vi "LM3Sxxxx_QEI_Config.vi"(8 "error in (no error)":errorcluster, 10 "Config Data":string[](array[string]), 11 "Interrupt Name":string) -> (0 "error out":errorcluster, 3 "Interrupt Configuration":string[](array[string]))   [LabVIEW 2011]
panel:
  in  "Phase error interrupt":bool
  in  "Direction change interrupt":bool
  in  "Index pulse interrupt":bool
  in  "Timer expire interrupt":bool
  in  "Period (ms)":u32=10
  in  "Velocity divider":u32(ring) items=["/1"=0, "/2"=64, "/4"=128, "/8"=192, "/16"=256, "/32"=320, "/64"=384, "/128"=448]
  in  "Enable":bool
  in  "Reset on index pulse":bool=TRUE
  in  "Maximum position":u32=1000
  in  "help":bool
  in  "Swap channel inputs":bool
  in  "Signal mode":u32(ring)=1 items=["Quadrature phase"=1, "Clock and direction"=0]
  in  "cancel":bool
  in  "ok":bool
  in  "Quadrature update mode":u32(ring)=1 items=["Capture A and B"=1, "Capture A only"=0]
  # "Input"
  # "Position"
  # "Velocity"
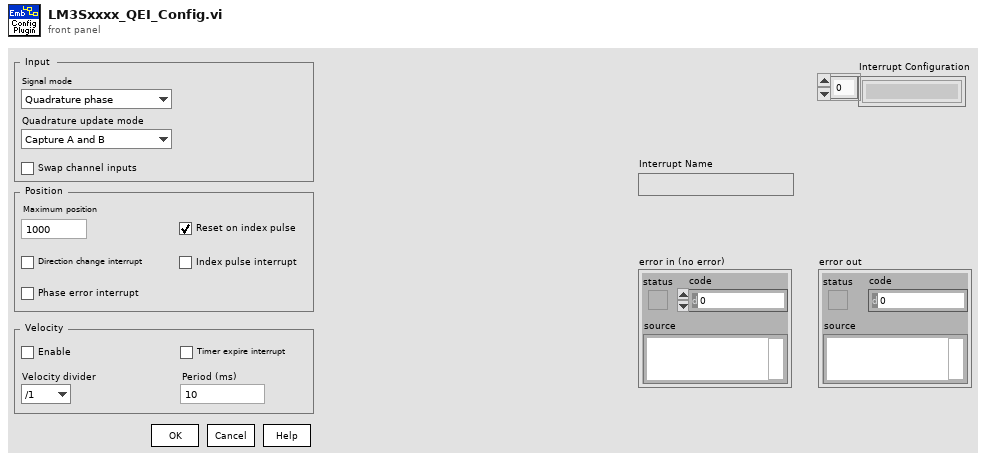
[diagram p1: front panel]
types:
  T1 = enum8{"Enabled", "Disabled", "Disabled and Grayed Out"}
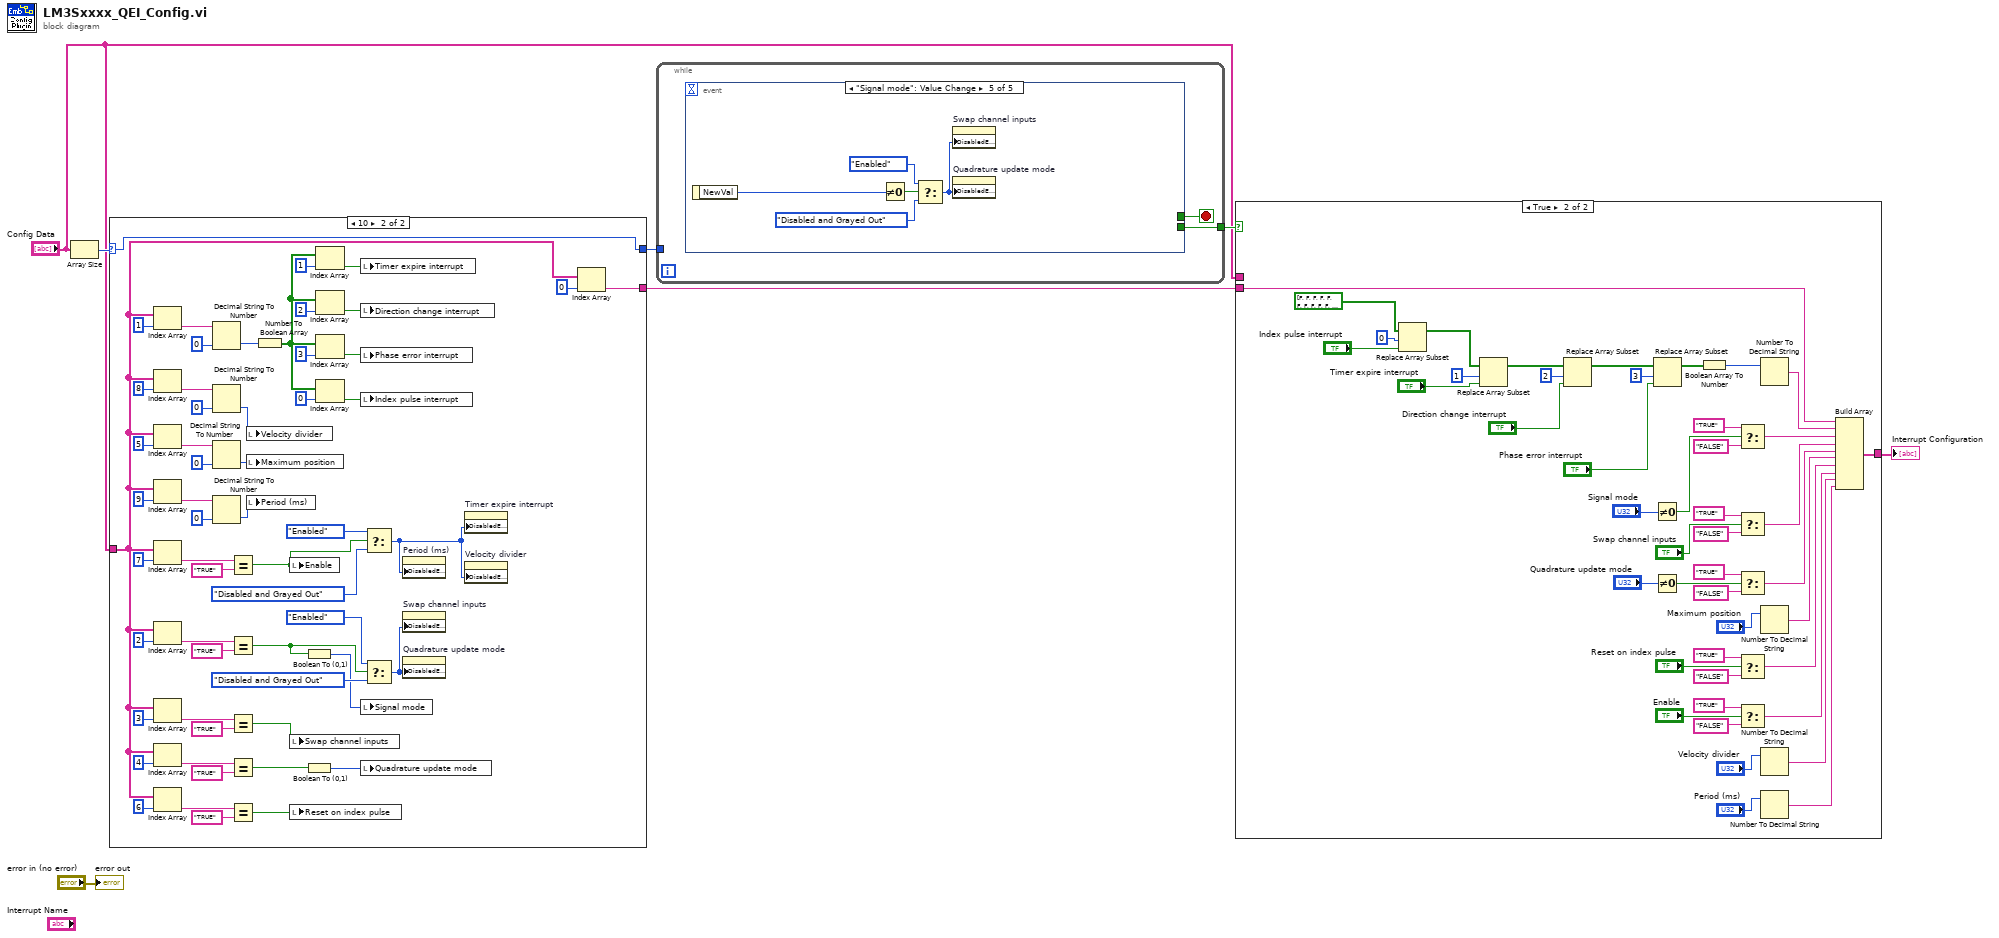
[diagram p0: block diagram]
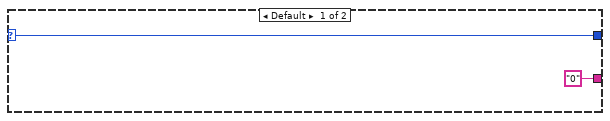
[diagram p2: hidden frame]
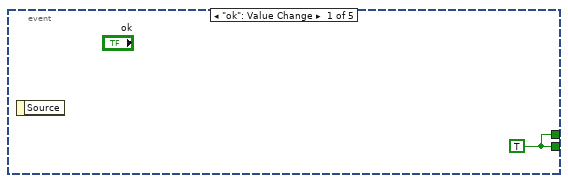
[diagram p4: hidden frame]
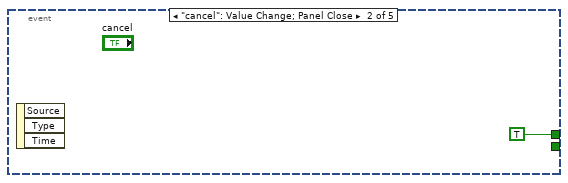
[diagram p5: hidden frame]
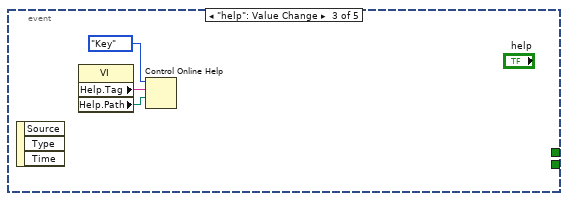
[diagram p6: hidden frame]
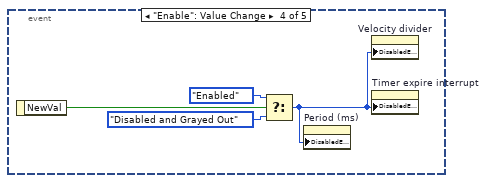
[diagram p7: hidden frame]
diagram:
  n1 = Array Size(array="Config Data") -> (size(s)=w4:i32)
  n2 = case shown="10" w4 {
    selector: w4 -> [w9 w66]
    tunnel: [w9 w66] -> w3
    tunnel: "Config Data" -> [_ w65]
    tunnel: ["0" ("String") w54] -> w2
    frame Default {
    }
    frame 10 {
      n3 = Index Array(array=w65, index=1) -> (element=w21:string)
      n4 = Index Array(array=w65, index=8) -> (element=w26:string)
      n5 = Index Array(array=w65, index=5) -> (element=w34:string)
      n6 = Index Array(array=w65, index=9) -> (element=w24:string)
      n7 = Index Array(array=w65, index=7) -> (element=w53:string)
      n8 = Index Array(array=w65, index=2) -> (element=w48:string)
      n9 = Index Array(array=w65, index=3) -> (element=w40:string)
      n10 = Index Array(array=w65, index=4) -> (element=w37:string)
      n11 = Index Array(array=w65, index=6) -> (element=w30:string)
      n12 = Decimal String To Number(string=w21, default (0L)=u32 0 ("default (0 I32)")) -> (number=w20:u32)  [unwired: 1 in, 1 out]
      n13 = Decimal String To Number(string=w26, default (0L)=u32 0 ("default (0 I32)")) -> (number=w25:u32)  [unwired: 1 in, 1 out]
      n14 = Decimal String To Number(string=w34, default (0L)=u32 0 ("default (0 I32)")) -> (number=w32:u32)  [unwired: 1 in, 1 out]
      n15 = Decimal String To Number(string=w24, default (0L)=u32 0 ("default (0 I32)")) -> (number=w23:u32)  [unwired: 1 in, 1 out]
      n16 = Equal?(x=w53, y="TRUE") -> (x = y?=w10:bool)
      n17 = Equal?(x=w48, y="TRUE") -> (x = y?=w46:bool)
      n18 = Equal?(x=w40, y="TRUE") -> (x = y?=w39:bool)
      n19 = Equal?(x=w37, y="TRUE") -> (x = y?=w36:bool)
      n20 = Equal?(x=w30, y="TRUE") -> (x = y?=w29:bool)
      n21 = local write "Velocity divider"(w25) -> ()
      n22 = local write "Maximum position"(w32) -> ()
      n23 = local write "Period (ms)"(w23) -> ()
      n24 = Number To Boolean Array(number=w20) -> (Boolean array=w19:bool[])
      n25 = local write "Enable"(w10) -> ()
      n26 = local write "Swap channel inputs"(w39) -> ()
      n27 = local write "Reset on index pulse"(w29) -> ()
      n28 = Boolean To (0,1)(Boolean=w46) -> (0, 1=w43:i16)
      n29 = Boolean To (0,1)(Boolean=w36) -> (0, 1=w35:i16)
      n30 = Index Array(array=w19, index=1) -> (element=w13:bool)
      n31 = Index Array(array=w19, index=2) -> (element=w12:bool)
      n32 = Index Array(array=w19, index=3) -> (element=w11:bool)
      n33 = Index Array(array=w19, index=0) -> (element=w14:bool)
      n34 = local write "Timer expire interrupt"(w13) -> ()
      n35 = local write "Direction change interrupt"(w12) -> ()
      n36 = local write "Phase error interrupt"(w11) -> ()
      n37 = local write "Index pulse interrupt"(w14) -> ()
      n38 = local write "Signal mode"(w43) -> ()
      n39 = local write "Quadrature update mode"(w35) -> ()
      n40 = Select(t=T1."Enabled" ("Disabled"), s=w10, f=T1."Disabled and Grayed Out") -> (s? t:f=w49:T1)
      n41 = Select(t=T1."Enabled" ("Disabled"), s=w46, f=T1."Disabled and Grayed Out") -> (s? t:f=w42:T1)
      n42 = property on="Period (ms)" class="DigNum (strict)"("DisabledEnum"=w49) -> ()  [unwired: 2 in, 2 out]
      n43 = property on="Swap channel inputs" class="Bool (strict)"("DisabledEnum"=w42) -> ()  [unwired: 2 in, 2 out]
      n44 = property on="Quadrature update mode" class="Ring (strict)"("DisabledEnum"=w42) -> ()  [unwired: 2 in, 2 out]
      n45 = property on="Timer expire interrupt" class="Bool (strict)"("DisabledEnum"=w49) -> ()  [unwired: 2 in, 2 out]
      n46 = property on="Velocity divider" class="Ring (strict)"("DisabledEnum"=w49) -> ()  [unwired: 2 in, 2 out]
      n47 = Index Array(array=w65, index=0) -> (element=w54:string)
    }
  }
  n48 = while {
    tunnel: [w67] -> w6
    tunnel: w3 -> [_]
    stop <- w68 stop-if-true
    n49 = event shown="[4] \"Signal mode\": Value Change" {
      selector: _ -> [_ _ _ _ _]
      dyn-events: _ -> [_ _ _ _ _]
      timeout: _ -> [_ _ _ _ _]
      tunnel: [w69 TRUE _ _ _] -> w68
      tunnel: [w69 _ _ _ _] -> w67
      event "ok": Value Change {
        w69 = TRUE
        n50 = event-data() -> ()  [unwired: 2 out]
      }
      event "cancel": Value Change; Panel Close {
        n51 = event-data() -> ()  [unwired: 4 out]
      }
      event "help": Value Change {
        n52 = event-data() -> ()  [unwired: 4 out]
        n53 = property class="VI"() -> ("Help.Tag"=w71:string, "Help.Path"=w72:path)  [unwired: 2 in, 2 out]
        n54 = Control Online Help(2:w72, 3:w71, 4:enum16{"Contents", "Key", "Close"}."Key" ("Operation")) -> ()  [unwired: 1 in, 1 out]
      }
      event "Enable": Value Change {
        n55 = event-data() -> ("NewVal"=w74:bool)  [unwired: 1 out]
        n56 = Select(t=T1."Enabled" ("Disabled"), s=w74, f=T1."Disabled and Grayed Out") -> (s? t:f=w77:T1)
        n57 = property on="Period (ms)" class="DigNum (strict)"("DisabledEnum"=w77) -> ()  [unwired: 2 in, 2 out]
        n58 = property on="Velocity divider" class="Ring (strict)"("DisabledEnum"=w77) -> ()  [unwired: 2 in, 2 out]
        n59 = property on="Timer expire interrupt" class="Bool (strict)"("DisabledEnum"=w77) -> ()  [unwired: 2 in, 2 out]
      }
      event "Signal mode": Value Change {
        n60 = event-data() -> ("NewVal"=w82:u32)  [unwired: 1 out]
        n61 = Not Equal To 0?(x=w82) -> (x != 0?=w78:bool)
        n62 = Select(t=T1."Enabled" ("Disabled"), s=w78, f=T1."Disabled and Grayed Out") -> (s? t:f=w81:T1)
        n63 = property on="Swap channel inputs" class="Bool (strict)"("DisabledEnum"=w81) -> ()  [unwired: 2 in, 2 out]
        n64 = property on="Quadrature update mode" class="Ring (strict)"("DisabledEnum"=w81) -> ()  [unwired: 2 in, 2 out]
      }
    }
  }
  n65 = case shown="True" w6 {
    tunnel: "Config Data" -> [w83 _]
    tunnel: [w83 w127] -> w5
    tunnel: w2 -> [_ w128]
    frame False {
    }
    frame True {
      n66 = Replace Array Subset(array=bool[] [FALSE, FALSE, FALSE, FALSE, FALSE, FALSE, FALSE, FALSE, FALSE, FALSE, FALSE, FALSE, FALSE, FALSE, FALSE, FALSE, FALSE, FALSE, FALSE, FALSE, FALSE, FALSE, FALSE, FALSE, FALSE, FALSE, FALSE, FALSE, FALSE, FALSE, FALSE, FALSE], new element="Index pulse interrupt", index=0) -> (w125:bool[])
      n67 = Replace Array Subset(array=w125, new element="Timer expire interrupt", index=1) -> (w124:bool[])
      n68 = Replace Array Subset(array=w124, new element="Direction change interrupt", index=2) -> (w123:bool[])
      n69 = Replace Array Subset(array=w123, new element="Phase error interrupt", index=3) -> (w122:bool[])
      n70 = Not Equal To 0?(x="Signal mode") -> (x != 0?=w110:bool)
      n71 = Not Equal To 0?(x="Quadrature update mode") -> (x != 0?=w104:bool)
      n72 = Boolean Array To Number(Boolean array=w122) -> (number=w121:u32)
      n73 = Select(t="TRUE", s=w110, f="FALSE") -> (s? t:f=w107:string)
      n74 = Select(t="TRUE", s="Swap channel inputs", f="FALSE") -> (s? t:f=w98:string)
      n75 = Select(t="TRUE", s=w104, f="FALSE") -> (s? t:f=w102:string)
      n76 = Select(t="TRUE", s="Reset on index pulse", f="FALSE") -> (s? t:f=w92:string)
      n77 = Select(t="TRUE", s="Enable", f="FALSE") -> (s? t:f=w88:string)
      n78 = Number To Decimal String(number=w121) -> (decimal integer string=w120:string)  [unwired: 1 in]
      n79 = Number To Decimal String(number="Maximum position") -> (decimal integer string=w96:string)  [unwired: 1 in]
      n80 = Number To Decimal String(number="Velocity divider") -> (decimal integer string=w86:string)  [unwired: 1 in]
      n81 = Number To Decimal String(number="Period (ms)") -> (decimal integer string=w84:string)  [unwired: 1 in]
      n82 = Build Array(w128, w120, w107, w98, w102, w96, w92, w88, w86, w84) -> (w127:string[])
    }
  }
  "Interrupt Configuration" <- w5
  "error out" <- "error in (no error)"
